vi "Generate Row Cells.vi"(0 "PDF Report":T31(xcontrol), 1 "Title format":T10={"Font"={"Name"="", "Size"=-1.0, "Color"=0, "Style"={"Bold"=TRUE, "Italic"=FALSE, "Underline"=FALSE, "Strikeout"=FALSE}}, "Align. and LS"={"Horizontal"=enum."CENTER", "Vertical"=enum."MIDDLE", "Line spacing"=enum."1.0"}}, 2 "Datas format":T10={"Font"={"Name"="", "Size"=-1.0, "Color"=0, "Style"={"Bold"=FALSE, "Italic"=FALSE, "Underline"=FALSE, "Strikeout"=FALSE}}, "Align. and LS"={"Horizontal"=enum."CENTER", "Vertical"=enum."MIDDLE", "Line spacing"=enum."1.0"}}, 7 "Custom Borders":T16={"Title Row Border"={"Line"={"Thickness"=1.0, "Color"=0}, "Column Borders [ ]"=[]}, "Datas Row Borders [ ]"=[]}, 11 "error in (no error)":errorcluster) -> (4 "PDF Report duplicate":T31(xcontrol), 6 "References":T3, 8 "Datas Row Cells [ ]":T9, 10 "Title Row Cells":T4={"Cell Cluster"={"Font Ref"=refnum, "Leading"=18.0, "Horizontal Aligment"=enum."JUSTIFY", "Vertical Alignment"=enum."BOTTOM"}, "PdfPCell [ ]"=[]}, 15 "error out":errorcluster)   [LabVIEW 2012]
doc: "Version 1.0\nDeveloped by Jean-Marc Simard\nCopyright © 2010, Exaprom Inc.\nAll rights reserved.\nLicense: BSD\n\nWith iTextSharp 4.1.6 (http://itextsharp.sourceforge.net)\nunder Mozilla Public License Version 1.1\n(http://www.mozilla.org/MPL/MPL-1.1.html)"
uses:
  Controls/PDF Report Xcontrol/PDF Report.xctl
  Controls/Row Border Title.ctl
  Controls/Cell Border.ctl
  Controls/Row Borders [ ] Datas.ctl
  Controls/Cell Properties Table.ctl
  Controls/Font cluster.ctl
  Controls/Font size.ctl
  Controls/Font color.ctl
  Controls/Texte alignement.ctl
  Controls/Cell Vertical alignment.ctl
  Controls/Line spacing.ctl
  Controls/Row PdfPCell [ ] Datas.ctl
  Controls/Cell Cluster.ctl
  C:/Users/MaxCorp/Documents/TopPerm - Base/DLL/itextsharp.dll
  DLL/itextsharp.dll
  Controls/Title Cells with refnum.ctl
  Controls/Cell Generic Format without Font.ctl
  Controls/Cell Generic Format.ctl
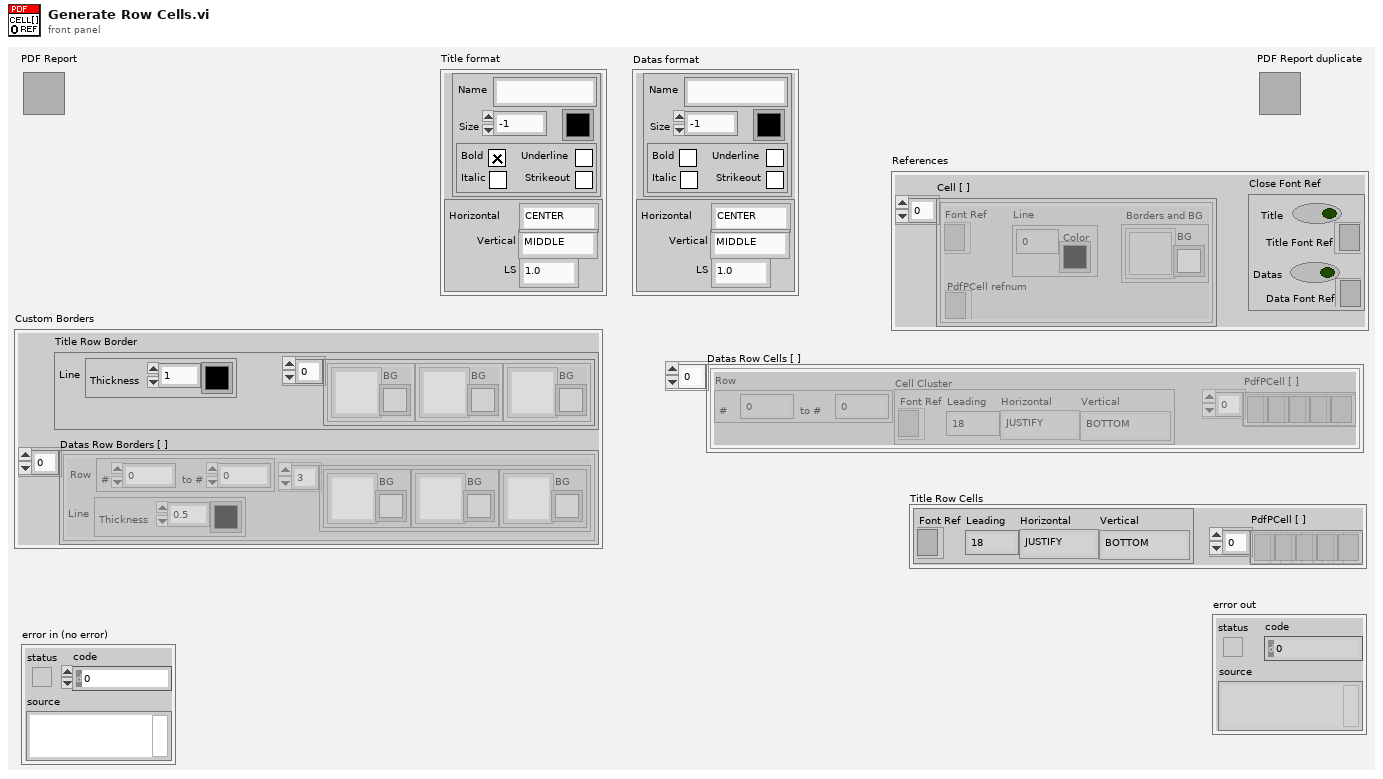
[diagram p1: front panel]
types:
  T1 = typedef "Cell Generic Format without Font.ctl" = cluster{"Font Ref":refnum<k24>, "Line":cluster{"Thickness":sgl, "Color":u32}, "Borders and BG":cluster{"Cell Border":T2, "BG":u32}, "PdfPCell refnum":refnum<k24>}
  T2 = typedef "Cell Border.ctl" = u16
  T3 = cluster{"Cell [ ]":T1[], "Close Font Ref":cluster{"Title":bool, "Title Font Ref":refnum<k24>, "Datas":bool, "Data Font Ref":refnum<k24>}}
  T4 = typedef "Title Cells with refnum.ctl" = cluster{"Cell Cluster":T5, "PdfPCell [ ]":refnum<k24>[]}
  T5 = typedef "Cell Cluster.ctl" = cluster{"Font Ref":refnum<k24>, "Leading":T6, "Horizontal Aligment":T7, "Vertical Alignment":T8}
  T6 = typedef "Font size.ctl" = sgl
  T7 = typedef "Texte alignement.ctl" = enum16{"Select", "CENTER", "JUSTIFY", "LEFT", "RIGHT"}
  T8 = typedef "Cell Vertical alignment.ctl" = enum16{"TOP", "MIDDLE", "BOTTOM"}
  T9 = typedef "Row PdfPCell [ ] Datas.ctl" = cluster{"Row":cluster{"#":i16, "to #":i16}, "Cell Cluster":T5, "PdfPCell [ ]":refnum<k24>[]}[]
  T10 = typedef "Cell Properties Table.ctl" = cluster{"Font":T11, "Align. and LS":cluster{"Horizontal":T7, "Vertical":T8, "Line spacing":T13}}
  T11 = typedef "Font cluster.ctl" = cluster{"Name":string, "Size":T6, "Color":T12, "Style":cluster{"Bold":bool, "Italic":bool, "Underline":bool, "Strikeout":bool}}
  T12 = typedef "Font color.ctl" = u32
  T13 = typedef "Line spacing.ctl" = enum16{"Select", "1.0", "1.5", "2.0"}
  T14 = typedef "Row Border Title.ctl" = cluster{"Line":cluster{"Thickness":sgl, "Color":u32}, "Column Borders [ ]":cluster{"Cell Border":T2, "BG":u32}[]}
  T15 = typedef "Row Borders [ ] Datas.ctl" = cluster{"Row":cluster{"#":i16, "to #":i16}, "Line":cluster{"Thickness":sgl, "Color":u32}, "Column Borders [ ]":cluster{"Cell Border":T2, "BG":u32}[]}[]
  T16 = cluster{"Title Row Border":T14, "Datas Row Borders [ ]":T15}
  T17 = typedef "Unit.ctl" = enum16{"inch", "mm"}
  T18 = typedef "Paragraphe cluster.ctl" = cluster{" Aligment":T7, "Line spacing":T13}
  T19 = typedef "Page dimensions.ctl" = cluster{"Start at page":i32, "Orientation":T20, "widht":sgl, "height":sgl, "Margin left":sgl, "Margin right":sgl, "Margin top":sgl, "Margin bottom":sgl}
  T20 = typedef "Page Orientation.ctl" = enum16{"Portrait", "Landscape"}
  T21 = typedef "Image or Table Caption.ctl" = cluster{"Caption":string, "Separator":string, "Position":enum16{"Above", "Below"}}
  T22 = typedef "Header Footer [ ].ctl" = T23[]
  T23 = typedef "Header Footer cluster.ctl" = cluster{"Start page":i32, "Type":T24, "Alignment":T25, "Vertical Alignement":T8, "Image (%)":sgl, "Page #":T26, "Text":string, "Path":string, "Font":T11, "Font refnum":refnum<k24>, "Line":cluster{"Line":T27, "Thickness (points)":sgl, "Colour":T12}}
  T24 = typedef "Header Footer Type.ctl" = enum16{"Select", "Text", "Text + hyperlink", "Page number", "Image", "Image + hyperlink"}
  T25 = typedef "Header footer horiz alignment.ctl" = enum16{"Left", "Center", "Right"}
  T26 = typedef "Page number.ctl" = cluster{"Text 1":string, "Text 2":string, "Text 3":string}
  T27 = typedef "Header Footer Line.ctl" = enum16{"No line", "Horizontal line"}
  T28 = typedef "Watermark cluster2.ctl" = cluster{"Show? (F)":bool, "Type":enum16{"Image", "Text"}, "Opacity (%)":sgl, "Rotate(°)":sgl, "Position":cluster{"Position":T29, "X":sgl, "Y":sgl}, "Image path":path, "Scaled(%)":sgl, "Image refnum":refnum<k24>, "Text":string, "Font":cluster{"Name":string, "Size":T6, "Color":T12}, "Font refnum":refnum<k24>, "Alignment":T25, "Automatic":bool}
  T29 = typedef "Watermark Position.ctl" = enum16{"Absolute", "Center (page)", "Center (text section)"}
  T30 = typedef "System Fonts.ctl" = cluster{"Font name [ ]":string[], "Font and file names [ ]":cluster{"Font name":string, "File name":string}[]}
  T31 = cluster{"Document":refnum<k24>, "Writer":refnum<k24>, "Default Font":refnum<k24>, "Default Font cluster":T11, "Path":path, "Unit (default = mm)":T17, "Paragraphe cluster":T18, "Pages dimensions [ ]":T19[], "Captions":cluster{"Image":T21, "Image counter":u16, "Table":T21, "Table counter":u16, "Font":T11}, "Header":T22, "Footer":T22, "Watermark ":T28, "Actual VI name":string, "System Fonts":T30}
  T32 = typedef "Cell Generic Format.ctl" = cluster{"Cell Text Format":T10, "Line":cluster{"Thickness":sgl, "Color":u32}, "Borders and BG":cluster{"Cell Border":T2, "BG":u32}, "PdfPCell refnum":refnum<k24>}
  T33 = cluster{cluster{"Font Ref":refnum<k24>, "Line":cluster{"Thickness":sgl, "Color":u32}, "Borders and BG":cluster{"Cell Border":T2, "BG":u32}, "Cell ref":refnum<k24>}[], cluster{"Close Font Ref":bool, "Font Ref":refnum<k24>, "Close Font Ref":bool, "Font Ref":refnum<k24>}}
  T34 = cluster{"Close Font Ref":bool, "Font Ref":refnum<k24>, "Close Font Ref":bool, "Font Ref":refnum<k24>}
  T35 = cluster{"Title format":T10, "Line":cluster{"Thickness":sgl, "Color":u32}, "Cluster 2":cluster{"Cell Border":T2, "BG":u32}, "PdfPCell refnum":refnum<k24>}
  T36 = cluster{"Datas format":T10, "Line":cluster{"Thickness":sgl, "Color":u32}, "Cluster 2":cluster{"Cell Border":T2, "BG":u32}, "PdfPCell refnum":refnum<k24>}
  T37 = cluster{"Cell Cluster":T5, "Line":cluster{"Thickness":sgl, "Color":u32}, "Borders and BG":cluster{"Cell Border":T2, "BG":u32}, "PdfPCell refnum":refnum<k24>}
  T38 = cluster{"Font Ref":refnum<k24>, "Line":cluster{"Thickness":sgl, "Color":u32}, "Borders and BG":cluster{"Cell Border":T2, "BG":u32}, "PdfP Cell ref":refnum<k24>}
  T39 = cluster{"Cell Cluster":T5, "Line":cluster{"Thickness":sgl, "Color":u32}, "Cluster 2":cluster{"Cell Border":T2, "BG":u32}, "PdfPCell refnum":refnum<k24>}
  T40 = cluster{"Font Ref":refnum<k24>, "Line":cluster{"Thickness":sgl, "Color":u32}, "Cluster 2":cluster{"Cell Border":T2, "BG":u32}, "PdfP Cell ref":refnum<k24>}
  T41 = cluster{"Font Ref":refnum<k24>, "Line":cluster{"Thickness":sgl, "Color":u32}, "Borders and BG":cluster{"Cell Border":T2, "BG":u32}, "PdfP Cell ref":refnum<k24>}[]
  T42 = cluster{cluster{"Font Ref":refnum<k24>, "Line":cluster{"Thickness":sgl, "Color":u32}, "Borders and BG":cluster{"Cell Border":T2, "BG":u32}, "PdfP Cell ref":refnum<k24>}[], cluster{"Close Font Ref":bool, "Font Ref":refnum<k24>, "Close Font Ref":bool, "Font Ref":refnum<k24>}}
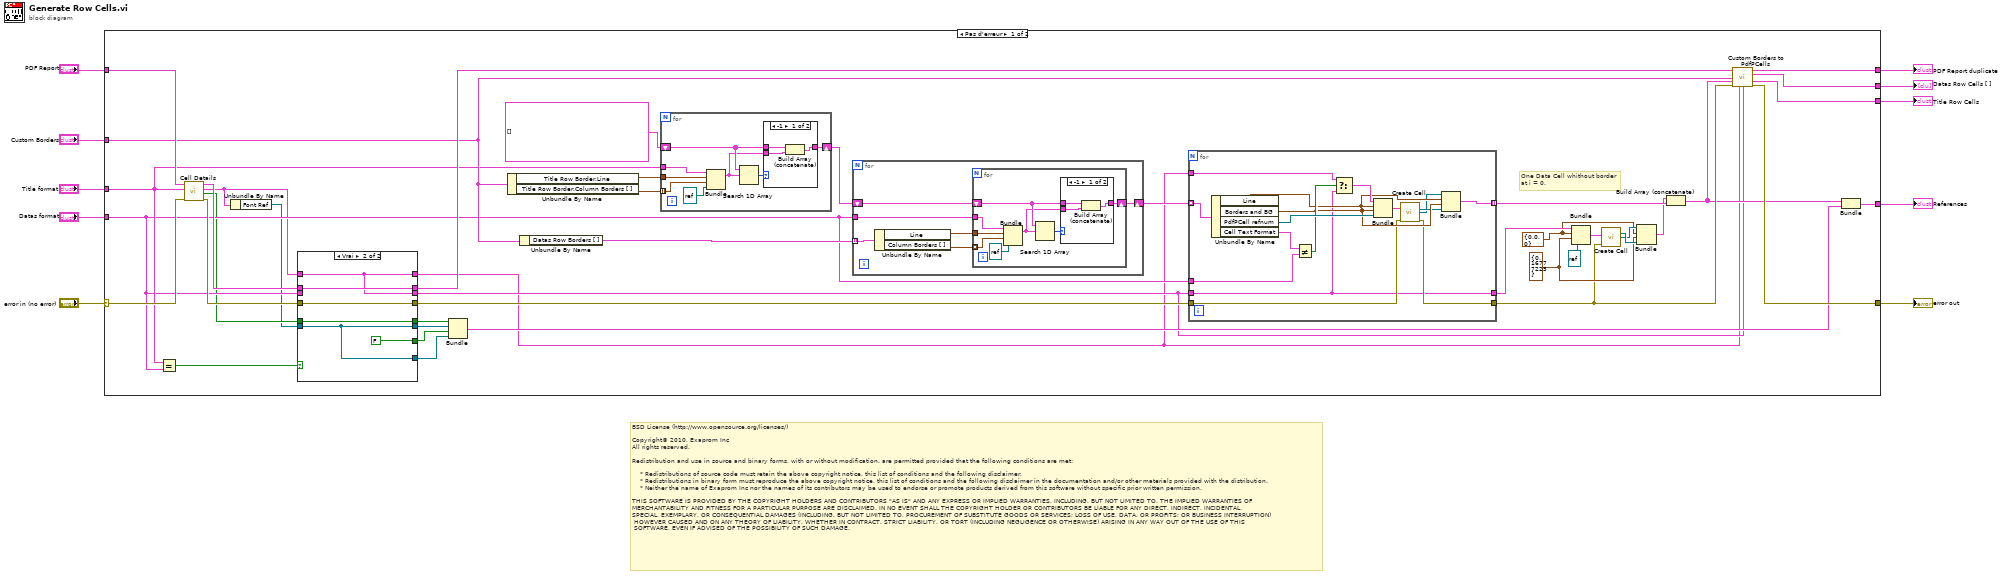
[diagram p0: block diagram]
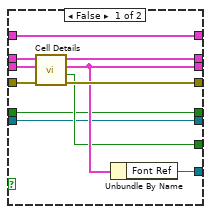
[diagram p2: hidden frame]
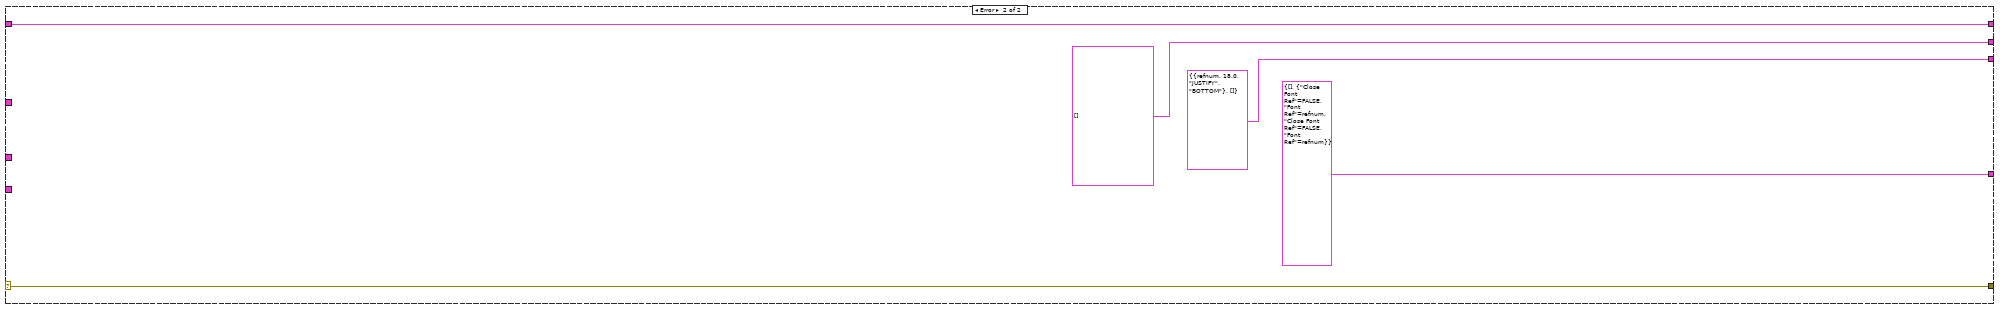
[diagram p5: hidden frame]
diagram:
  # "BSD License (http://www.opensource.org/licenses/)\n\nCopyright© 2010, Exaprom Inc\nAll rights reserved.\n\nRedistribution and use in source and binary forms, with or without modification, are permitted provided that the following conditions are met:\n\n    * Redistributions of source code must retain the above copyright notice, this list of conditions and the following disclaimer.\n    * Redistributions in binary form must reproduce the above copyright notice, this list of conditions and the following disclaimer in the documentation and/or other materials provided with the distribution.\n    * Neither the name of Exaprom Inc nor the names of its contributors may be used to endorse or promote products derived from this software without specific prior written permission.\n\nTHIS SOFTWARE IS PROVIDED BY THE COPYRIGHT HOLDERS AND CONTRIBUTORS \"AS IS\" AND ANY EXPRESS OR IMPLIED WARRANTIES, INCLUDING, BUT NOT LIMITED TO, THE IMPLIED WARRANTIES OF \nMERCHANTABILITY AND FITNESS FOR A PARTICULAR PURPOSE ARE DISCLAIMED. IN NO EVENT SHALL THE COPYRIGHT HOLDER OR CONTRIBUTORS BE LIABLE FOR ANY DIRECT, INDIRECT, INCIDENTAL,\nSPECIAL, EXEMPLARY, OR CONSEQUENTIAL DAMAGES (INCLUDING, BUT NOT LIMITED TO, PROCUREMENT OF SUBSTITUTE GOODS OR SERVICES; LOSS OF USE, DATA, OR PROFITS; OR BUSINESS INTERRUPTION)\n HOWEVER CAUSED AND ON ANY THEORY OF LIABILITY, WHETHER IN CONTRACT, STRICT LIABILITY, OR TORT (INCLUDING NEGLIGENCE OR OTHERWISE) ARISING IN ANY WAY OUT OF THE USE OF THIS\n SOFTWARE, EVEN IF ADVISED OF THE POSSIBILITY OF SUCH DAMAGE."
  n1 = case shown="Pas d'erreur" "error in (no error)" {
    selector: "error in (no error)" -> [w46 w120]
    tunnel: "PDF Report" -> [w48 w119]
    tunnel: [w31 w119] -> w10
    tunnel: [w29 w120] -> w9
    tunnel: "Custom Borders" -> [w30 _]
    tunnel: "Title format" -> [w19 _]
    tunnel: "Datas format" -> [w18 _]
    tunnel: [w27 T9 [] ("Datas Row Cells [ ]")] -> w4
    tunnel: [w26 T4 {"Cell Cluster"={"Font Ref"=refnum, "Leading"=18.0, "Horizontal Aligment"=enum."JUSTIFY", "Vertical Alignment"=enum."BOTTOM"}, "PdfPCell [ ]"=[]} ("Title Row Cells")] -> w3
    tunnel: [w24 T33 {[], {"Close Font Ref"=FALSE, "Font Ref"=refnum, "Close Font Ref"=FALSE, "Font Ref"=refnum}}] -> w1
    frame No Error {
      w33 = cluster{"Cell Border":T2, "BG":u32} {"Cell Border"=0, "BG"=16777225} ("Cluster 2")
      w34 = cluster{"Thickness":sgl, "Color":u32} {"Thickness"=0.0, "Color"=0} ("Line")
      # "One Data Cell whithout border\nat i = 0."
      n2 = Equal?(x=w19, y=w18) -> (x = y?=w17:bool)
      n3 = call "Cell Details.vi"("error in (no error)"=w46, "Cell format"=w19, "PDF Report"=w48) -> ("error out"=w47:errorcluster, "Close Font Ref"=w15:bool, "Cell Cluster"=w12:T5, "PDF Report duplicate"=w49:T31)  [unwired: 5 out]
      n4 = Unbundle By Name(w12) -> ("Font Ref"=w13:refnum<k24>)
      n5 = case shown="Vrai" w17 {
        tunnel: w49 -> [w63 w66]
        tunnel: w47 -> [w62 w65]
        tunnel: [w61 w65] -> w42
        tunnel: [w60 w66] -> w32
        tunnel: [w59 w64] -> w22
        tunnel: [w58 FALSE ("Close Font Ref")] -> w21
        tunnel: [w57 w68] -> w20
        tunnel: w18 -> [w56 _]
        tunnel: [w55 w69] -> w16
        tunnel: w15 -> [w55 w69]
        tunnel: [w54 w68] -> w14
        tunnel: w13 -> [w54 w68]
        tunnel: w12 -> [w53 w64]
        tunnel: [w53 w64] -> w11
        frame False {
          n6 = call "Cell Details.vi"("error in (no error)"=w62, "Cell format"=w56, "PDF Report"=w63) -> ("error out"=w61:errorcluster, "Close Font Ref"=w58:bool, "Cell Cluster"=w59:T5, "PDF Report duplicate"=w60:T31)  [unwired: 5 out]
          n7 = Unbundle By Name(w59) -> ("Font Ref"=w57:refnum<k24>)
        }
        frame True {
        }
      }
      n8 = Bundle("Close Font Ref"=w16, "Font Ref"=w14, "Close Font Ref"=w21, "Font Ref"=w20) -> (w23:T34)  [unwired: 1 out]
      n9 = Unbundle By Name(w30) -> ("Title Row Border.Line"=w51:cluster{"Thickness":sgl, "Color":u32}, "Title Row Border.Column Borders [ ]"=w52:cluster{"Cell Border":T2, "BG":u32}[])
      n10 = Unbundle By Name(w30) -> ("Datas Row Borders [ ]"=w50:T15)
      n11 = for {
        tunnel: w52 -> [w110] mode=indexing
        shift-right: [w108] -> w45
        shift-left: T32[] [] -> [w107]
        tunnel: w51 -> [w111]
        tunnel: w19 -> [w104]
        n12 = Bundle("Title format"=w104, "Line"=w111, "Cluster 2"=w110, "PdfPCell refnum"=refnum<k24> refnum) -> (w106:T35)  [unwired: 1 out]
        n13 = Search 1D Array(1D array=w107, element=w106) -> (index of element=w109:i32)  [unwired: 1 out]
        n14 = case shown="-1" w109 {
          tunnel: [w112 w115] -> w108
          tunnel: w107 -> [w114 w115]
          tunnel: w106 -> [w113 _]
          frame -1 {
            n15 = Build Array (concatenate)(w114, w113) -> (w112:T32[])
          }
          frame 0.., Default {
          }
        }
      }
      n16 = for {
        tunnel: w50 -> [w91] mode=indexing
        shift-right: [w86] -> w44
        shift-left: w45 -> [w88]
        tunnel: w18 -> [w87]
        n17 = Unbundle By Name(w91) -> ("Line"=w89:cluster{"Thickness":sgl, "Color":u32}, "Column Borders [ ]"=w90:cluster{"Cell Border":T2, "BG":u32}[])
        n18 = for {
          tunnel: w90 -> [w97] mode=indexing
          shift-right: [w95] -> w86
          shift-left: w88 -> [w94]
          tunnel: w89 -> [w98]
          tunnel: w87 -> [w99]
          n19 = Bundle("Datas format"=w99, "Line"=w98, "Cluster 2"=w97, "PdfPCell refnum"=refnum<k24> refnum) -> (w93:T36)  [unwired: 1 out]
          n20 = Search 1D Array(1D array=w94, element=w93) -> (index of element=w96:i32)  [unwired: 1 out]
          n21 = case shown="-1" w96 {
            tunnel: [w100 w103] -> w95
            tunnel: w94 -> [w102 w103]
            tunnel: w93 -> [w101 _]
            frame -1 {
              n22 = Build Array (concatenate)(w102, w101) -> (w100:T32[])
            }
            frame 0.., Default {
            }
          }
        }
      }
      n23 = for {
        tunnel: w44 -> [w74] mode=indexing
        tunnel: w18 -> [w84]
        tunnel: w11 -> [w83]
        tunnel: w22 -> [w70]
        tunnel: [w75] -> w43 mode=indexing
        tunnel: w42 -> [w73]
        tunnel: [w72] -> w28
        tunnel: [w70] -> w39
        n24 = Unbundle By Name(w74) -> ("Line"=w78:cluster{"Thickness":sgl, "Color":u32}, "Borders and BG"=w77:cluster{"Cell Border":T2, "BG":u32}, "PdfPCell refnum"=w81:refnum<k24>, "Cell Text Format"=w85:T10)
        n25 = Not Equal?(x=w85, y=w84) -> (x != y?=w80:bool)
        n26 = Select(t=w83, s=w80, f=w70) -> (s? t:f=w82:T5)
        n27 = Bundle("Cell Cluster"=w82, "Line"=w78, "Borders and BG"=w77, "PdfPCell refnum"=w81) -> (w79:T37)  [unwired: 1 out]
        n28 = call "Create Cell.vi"("Cell Generic Format"=w79, "error in (no error)"=w73) -> ("PdfP Cell ref"=w76:refnum<k24>, "Font Ref"=w71:refnum<k24>, "error out"=w72:errorcluster)  [unwired: 11 out]
        n29 = Bundle("Font Ref"=w71, "Line"=w78, "Borders and BG"=w77, "PdfP Cell ref"=w76) -> (w75:T38)  [unwired: 1 out]
      }
      n30 = Bundle("Cell Cluster"=w39, "Line"=w34, "Cluster 2"=w33, "PdfPCell refnum"=refnum<k24> refnum) -> (w40:T39)  [unwired: 1 out]
      n31 = call "Create Cell.vi"("Cell Generic Format"=w40, "error in (no error)"=w28) -> ("PdfP Cell ref"=w37:refnum<k24>, "Font Ref"=w36:refnum<k24>)  [unwired: 12 out]
      n32 = Bundle("Font Ref"=w36, "Line"=w34, "Cluster 2"=w33, "PdfP Cell ref"=w37) -> (w35:T40)  [unwired: 1 out]
      n33 = Build Array (concatenate)(w35, w43) -> (w25:T41)
      n34 = call "Custom Borders to PdfPCells.vi"("PDF Report"=w32, "Custom Borders"=w30, "Cell [ ]"=w25, "error in (no error)"=w28, "Title format"=w11, "Data Format"=w22) -> ("PDF Report duplicate"=w31:T31, "Datas Row Cells [ ]"=w27:T9, "Title Row Cells"=w26:T4, "error out"=w29:errorcluster)  [unwired: 6 out]
      n35 = Bundle(w25, w23) -> (w24:T42)  [unwired: 1 out]
    }
    frame Error {
    }
  }
  "PDF Report duplicate" <- w10
  "error out" <- w9
  "Title Row Cells" <- w3
  "Datas Row Cells [ ]" <- w4
  "References" <- w1
